vi "Capture.vi"() -> ()   [LabVIEW 2012]
uses:
  <vilib>/userdefined/High Color/IMAQdx.ctl
  <vilib>/vision/driver/NI_Vision_Acquisition_Software.lvlib
panel:
  out "error out":errorcluster
  out "Image":T1(plugin-control)
  out "error out 2":errorcluster
  in  "error in (no error)":errorcluster caption="错误输入（无错误）"
  in  "停止":bool
  in  "error in":errorcluster
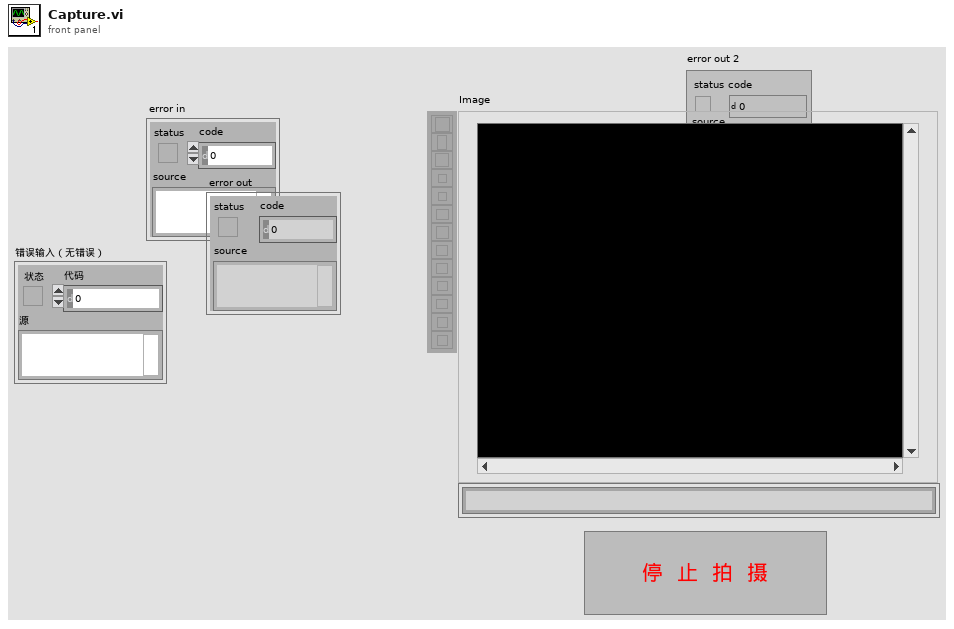
[diagram p1: front panel]
types:
  T1 = typedef "IMAQ Image.ctl" = refnum<image>
  T2 = typedef "IMAQdx.ctl" = refnum<k21>
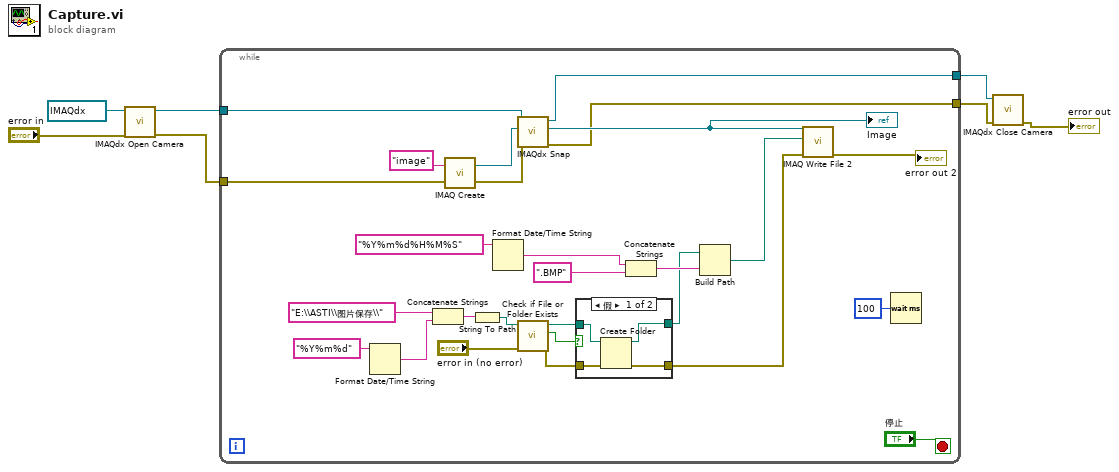
[diagram p0: block diagram]
diagram:
  n1 = call <vilib>:"IMAQdx Open Camera.vi"("error in"="error in", "Session In"=T2 "cam0") -> ("error out"=w4:errorcluster, "Session Out"=w5:T2)  [unwired: 8 in]
  n2 = while {
    tunnel: w5 -> [w34]
    tunnel: w4 -> [w32]
    tunnel: [w10] -> w3
    tunnel: [w9] -> w2
    stop <- "停止" stop-if-true
    n3 = Format Date/Time String(time format string (%c)="%Y%m%d" ("时间格式字符串(%c)")) -> (date/time string=w21:string)  [unwired: 2 in]
    n4 = Concatenate Strings("E:\\ASTI\\图片保存\\" ("字符串"), w21) -> (w20:string)
    n5 = call "IMAQ Create"("Image Name"="image", "error in (no error)"=w32) -> ("New Image"=w33:T1, "error out"=w31:errorcluster)  [unwired: 3 in]
    n6 = String To Path(string=w20) -> (path=w19:path)
    n7 = Format Date/Time String ("格式化日期/时间字符串")(time format string (%c)="%Y%m%d%H%M%S" ("时间格式字符串(%c)")) -> (date/time string=w27:string)  [unwired: 2 in]
    n8 = call <vilib>:"IMAQdx Snap.vi"("error in"=w31, "Image In"=w33, "Session In"=w34) -> ("error out"=w9:errorcluster, "Image Out"=w28:T1, "Session Out"=w10:T2)  [unwired: 6 in]
    "Image" <- w28
    n9 = call <vilib>:"Check if File or Folder Exists.vi"("error in (no error)"="error in (no error)", "path"=w19) -> ("error out"=w16:errorcluster, "file or folder exists?"=w18:bool, "dup path"=w17:path)  [unwired: 7 in]
    n10 = case shown="假" w18 {
      tunnel: w17 -> [w38 w40]
      tunnel: w16 -> [w37 w39]
      tunnel: [w36 w40] -> w12
      tunnel: [w35 w39] -> w15
      frame False {
        n11 = Create Folder(path (use dialog)=w38, error in=w37) -> (created path=w36:path, error out=w35:errorcluster)  [unwired: 1 in, 1 out]
      }
      frame True {
      }
    }
    n12 = Concatenate Strings(w27, ".BMP" ("字符串")) -> (w25:string)
    n13 = Build Path ("创建路径")(base path=w12, name or relative path=w25) -> (appended path=w30:path)
    n14 = call-poly "IMAQ Write File 2"("error in (no error)"=w15, "File Path"=w30, "Image"=w28) -> ("error out"=→"error out 2":errorcluster)  [unwired: 7 in, 1 out]
    n15 = Wait (ms)(milliseconds to wait=u32 100 ("等待时间（毫秒）")) -> ()  [unwired: 1 out]
  }
  n16 = call <vilib>:"IMAQdx Close Camera.vi"("error in"=w2, "Session In"=w3) -> ("error out"=→"error out":errorcluster)  [unwired: 9 in]
